vi "3.11-Create rotation Matrix.vi"(1 "Radians":dbl) -> (0 "appended array":dbl[][](array[numeric]))   [LabVIEW 2011]
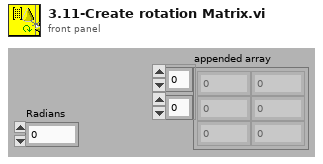
[diagram p1: front panel]
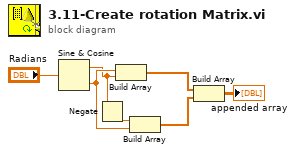
[diagram p0: block diagram]
diagram:
  n1 = Sine & Cosine(0:"Radians") -> (1:w5:dbl, 2:w6:dbl)
  n2 = Negate(x=w5) -> (-x=w4:dbl)
  n3 = Build Array(w6, w5) -> (w3:dbl[])
  n4 = Build Array(w4, w6) -> (w2:dbl[])
  n5 = Build Array(w3, w2) -> (→"appended array":dbl[][])
